vi "Write UI State.vi"(8 "error in (no error)":errorcluster, 10 "UI State":T1=enum."Embedded", 11 "EmbeddedSMO in":refnum<class "SMO.UI.Embedded.lvclass">) -> (0 "error out":errorcluster, 3 "EmbeddedSMO out":refnum<class "SMO.UI.Embedded.lvclass">)   [LabVIEW 2019, in "SMO.UI.Embedded.lvclass"]
uses:
  SMO.UI.Embedded.lvclass
  Typedefs/UI State.ctl
  SMO.UI.Embedded.lvclass/SMO.UI.Embedded.ctl
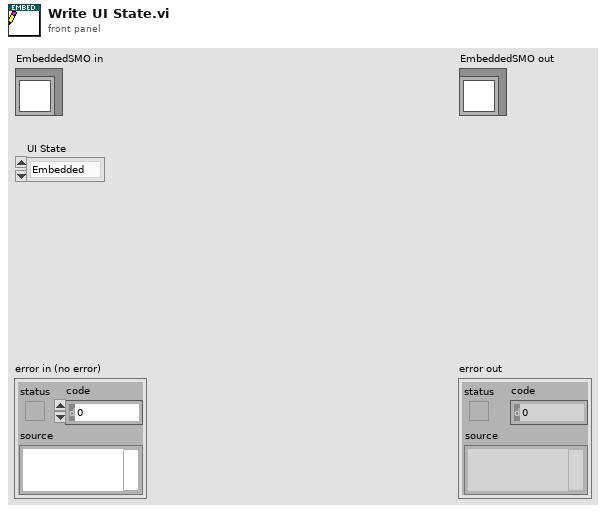
[diagram p1: front panel]
types:
  T1 = typedef "SMO.UI.Embedded.lvclass/UI State.ctl" = enum16{"unknown", "Opened", "Embedded", "Closed"}
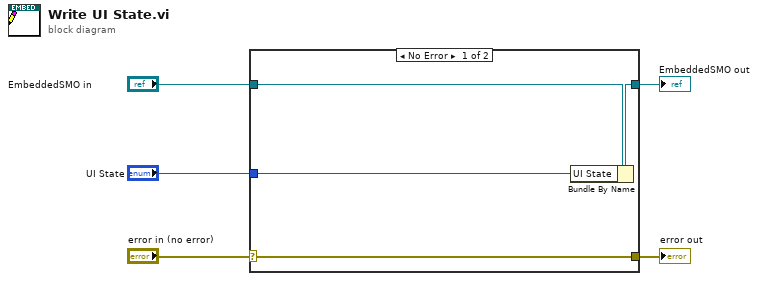
[diagram p0: block diagram]
diagram:
  n1 = case shown="No Error" "error in (no error)" {
    selector: "error in (no error)" -> [w9 w10]
    tunnel: [w9 w10] -> w4
    tunnel: [w7 w11] -> w2
    tunnel: "EmbeddedSMO in" -> [w8 w11]
    tunnel: "UI State" -> [w6 _]
    frame No Error {
      n2 = Bundle By Name(cluster=w8, "UI State"=w6) -> (w7:refnum<class "SMO.UI.Embedded.lvclass">)
    }
    frame Error {
    }
  }
  "error out" <- w4
  "EmbeddedSMO out" <- w2
